vi "Setup Statically-Linked subWorkers.vi"(8 "error in":errorcluster, 11 "Device Manager in":refnum<class "Device Manager.lvclass">) -> (0 "error out":errorcluster, 3 "Device Manager out":refnum<class "Device Manager.lvclass">)   [LabVIEW 2017, in "Device Manager.lvclass"]
doc: "This VI performs a setup of all the statically-linked subWorkers that belong to the Worker that owns this VI. This VI must be called <b>before</b> any statically-linked subWorkers are called."
uses:
  Device Manager.lvclass
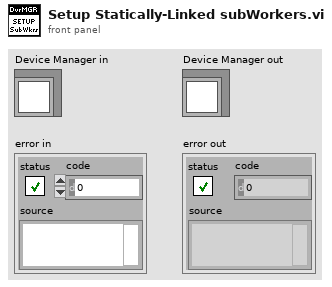
[diagram p1: front panel]
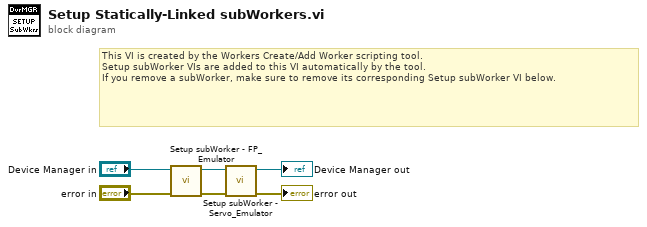
[diagram p0: block diagram]
diagram:
  # "This VI is created by the Workers Create/Add Worker scripting tool.\nSetup subWorker VIs are added to this VI automatically by the tool.\nIf you remove a subWorker, make sure to remove its corresponding Setup subWorker VI below."
  n1 = call "Setup subWorker - FP_Emulator.vi"("error in"="error in", "Device Manager in"="Device Manager in") -> ("error out"=w5:errorcluster, "Device Manager out"=w2:refnum<class "Device Manager.lvclass">)  [unwired: 8 in]
  n2 = call "Setup subWorker - Servo_Emulator.vi"("error in"=w5, "Device Manager in"=w2) -> ("error out"=→"error out":errorcluster, "Device Manager out"=→"Device Manager out":refnum<class "Device Manager.lvclass">)  [unwired: 8 in]
